vi "ThingSpeak.vi"() -> ()   [LabVIEW 2020]
uses:
  <vilib>/httpClient/POSTBuffer.vi
  <vilib>/httpClient/LabVIEWHTTPClient.lvlib
panel:
  in  "stop":bool
  out "error out":errorcluster
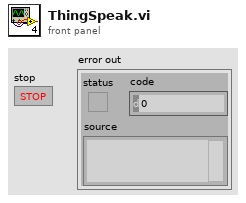
[diagram p1: front panel]
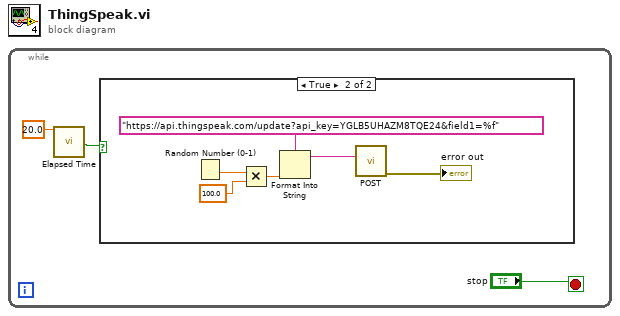
[diagram p0: block diagram]
diagram:
  n1 = while {
    stop <- "stop" stop-if-true
    n2 = call "Elapsed Time"("Time Target (s)"=20.0) -> ("Time has Elapsed"=w1:bool)  [unwired: 11 in, 7 out]
    n3 = case shown="True" w1 {
      frame False {
      }
      frame True {
        n4 = Random Number (0-1)() -> (number: 0 to 1=w9:dbl)
        n5 = Multiply(x=w9, y=100.0) -> (x*y=w7:dbl)
        n6 = Format Into String(format string="https://api.thingspeak.com/update?api_key=YGLB5UHAZM8TQE24&field1=%f", w7) -> (resulting string=w5:string)  [unwired: 2 in, 1 out]
        n7 = call-poly <vilib>:"POST.vi"("url"=w5) -> ("error out"=→"error out":errorcluster)  [unwired: 11 in, 3 out]
      }
    }
  }
